vi "Sudoku Solver.vi"(10 "Board":i32[][](array[numeric])=[[0, 0, 0, 0, 0, 0, 0, 0, 0], [0, 0, 0, 0, 0, 0, 0, 0, 0], [0, 0, 0, 0, 0, 0, 0, 0, 0], [0, 0, 0, 0, 0, 0, 0, 0, 0], [0, 0, 0, 0, 0, 0, 0, 0, 0], [0, 0, 0, 0, 0, 0, 0, 0, 0], [0, 0, 0, 0, 0, 0, 0, 0, 0], [0, 0, 0, 0, 0, 0, 0, 0, 0], [0, 0, 0, 0, 0, 0, 0, 0, 0]]) -> (1 "Solved":bool=TRUE, 3 "Sudoku Solution":i32[][](array[numeric])=[[4, 3, 5, 2, 6, 9, 7, 8, 1], [6, 8, 2, 5, 7, 1, 4, 9, 3], [1, 9, 7, 8, 3, 4, 5, 6, 2], [8, 2, 6, 1, 9, 5, 3, 4, 7], [3, 7, 4, 6, 8, 2, 9, 1, 5], [9, 5, 1, 7, 4, 3, 6, 2, 8], [5, 1, 9, 3, 2, 6, 8, 7, 4], [2, 4, 8, 9, 5, 7, 1, 3, 6], [7, 6, 3, 4, 1, 8, 2, 5, 9]])   [LabVIEW 2023]
doc: "Main VI of Sudoku Solver. \n\nInputs\n- Board: Input of Board Configuration\n- Current Cell: Row and Column of Current Cell\n\nOutputs\n- Sudoku Solution: Current Board Configuration\n- Solved: TRUE if Sudoku is solved"
panel:
  # "Instructions:\n1. Input your Sudoku in \"Board\". \"0\" represents empty cells.\n2. Run VI to solve the Sudoku"
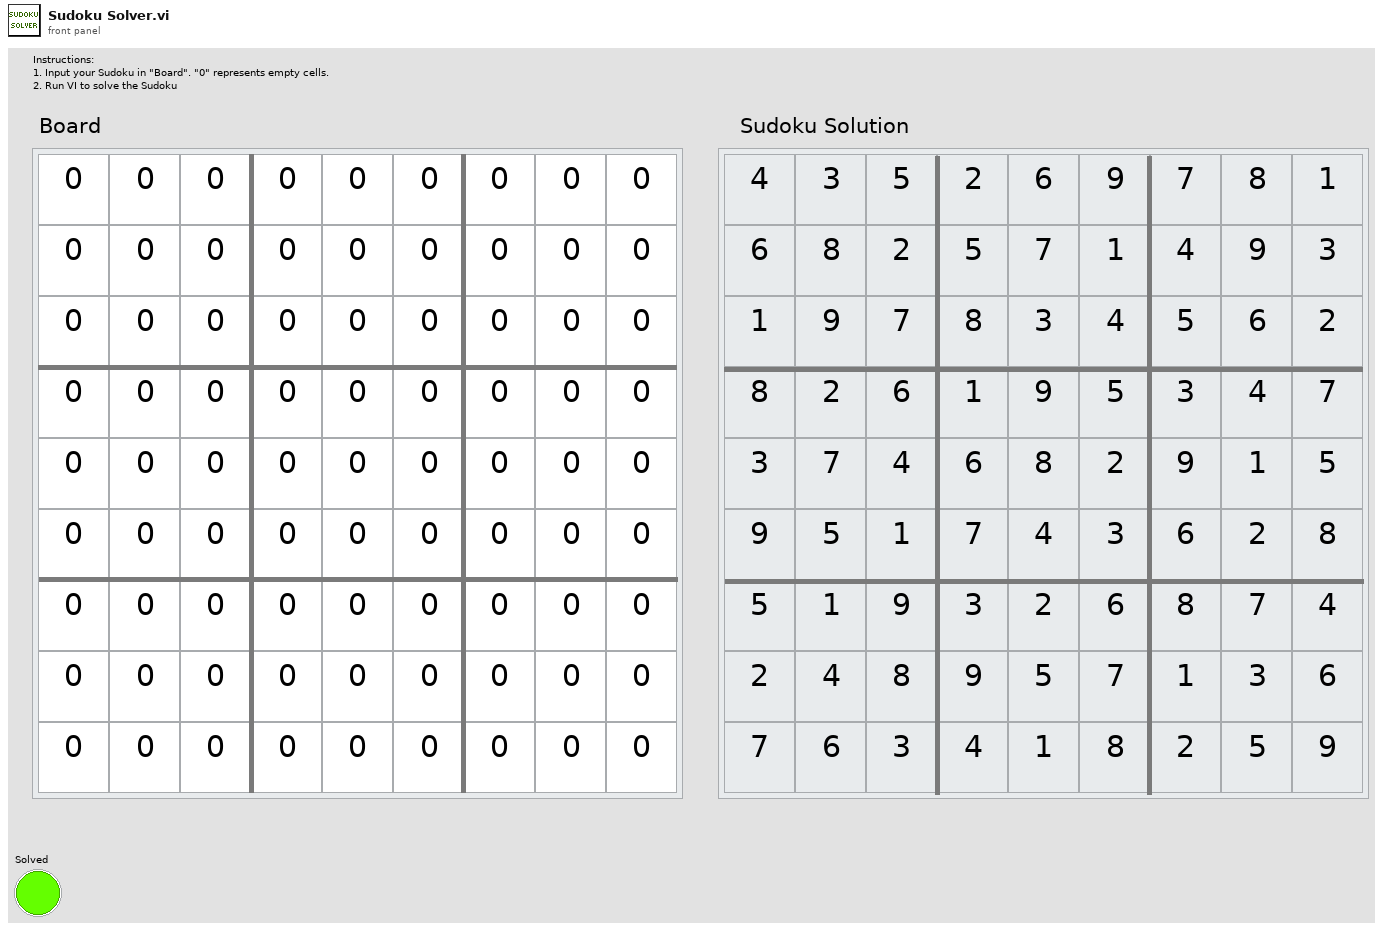
[diagram p1: front panel]
types:
  T1 = typedef "CurrentCell.ctl" = cluster{"Row":i32, "Column":i32}
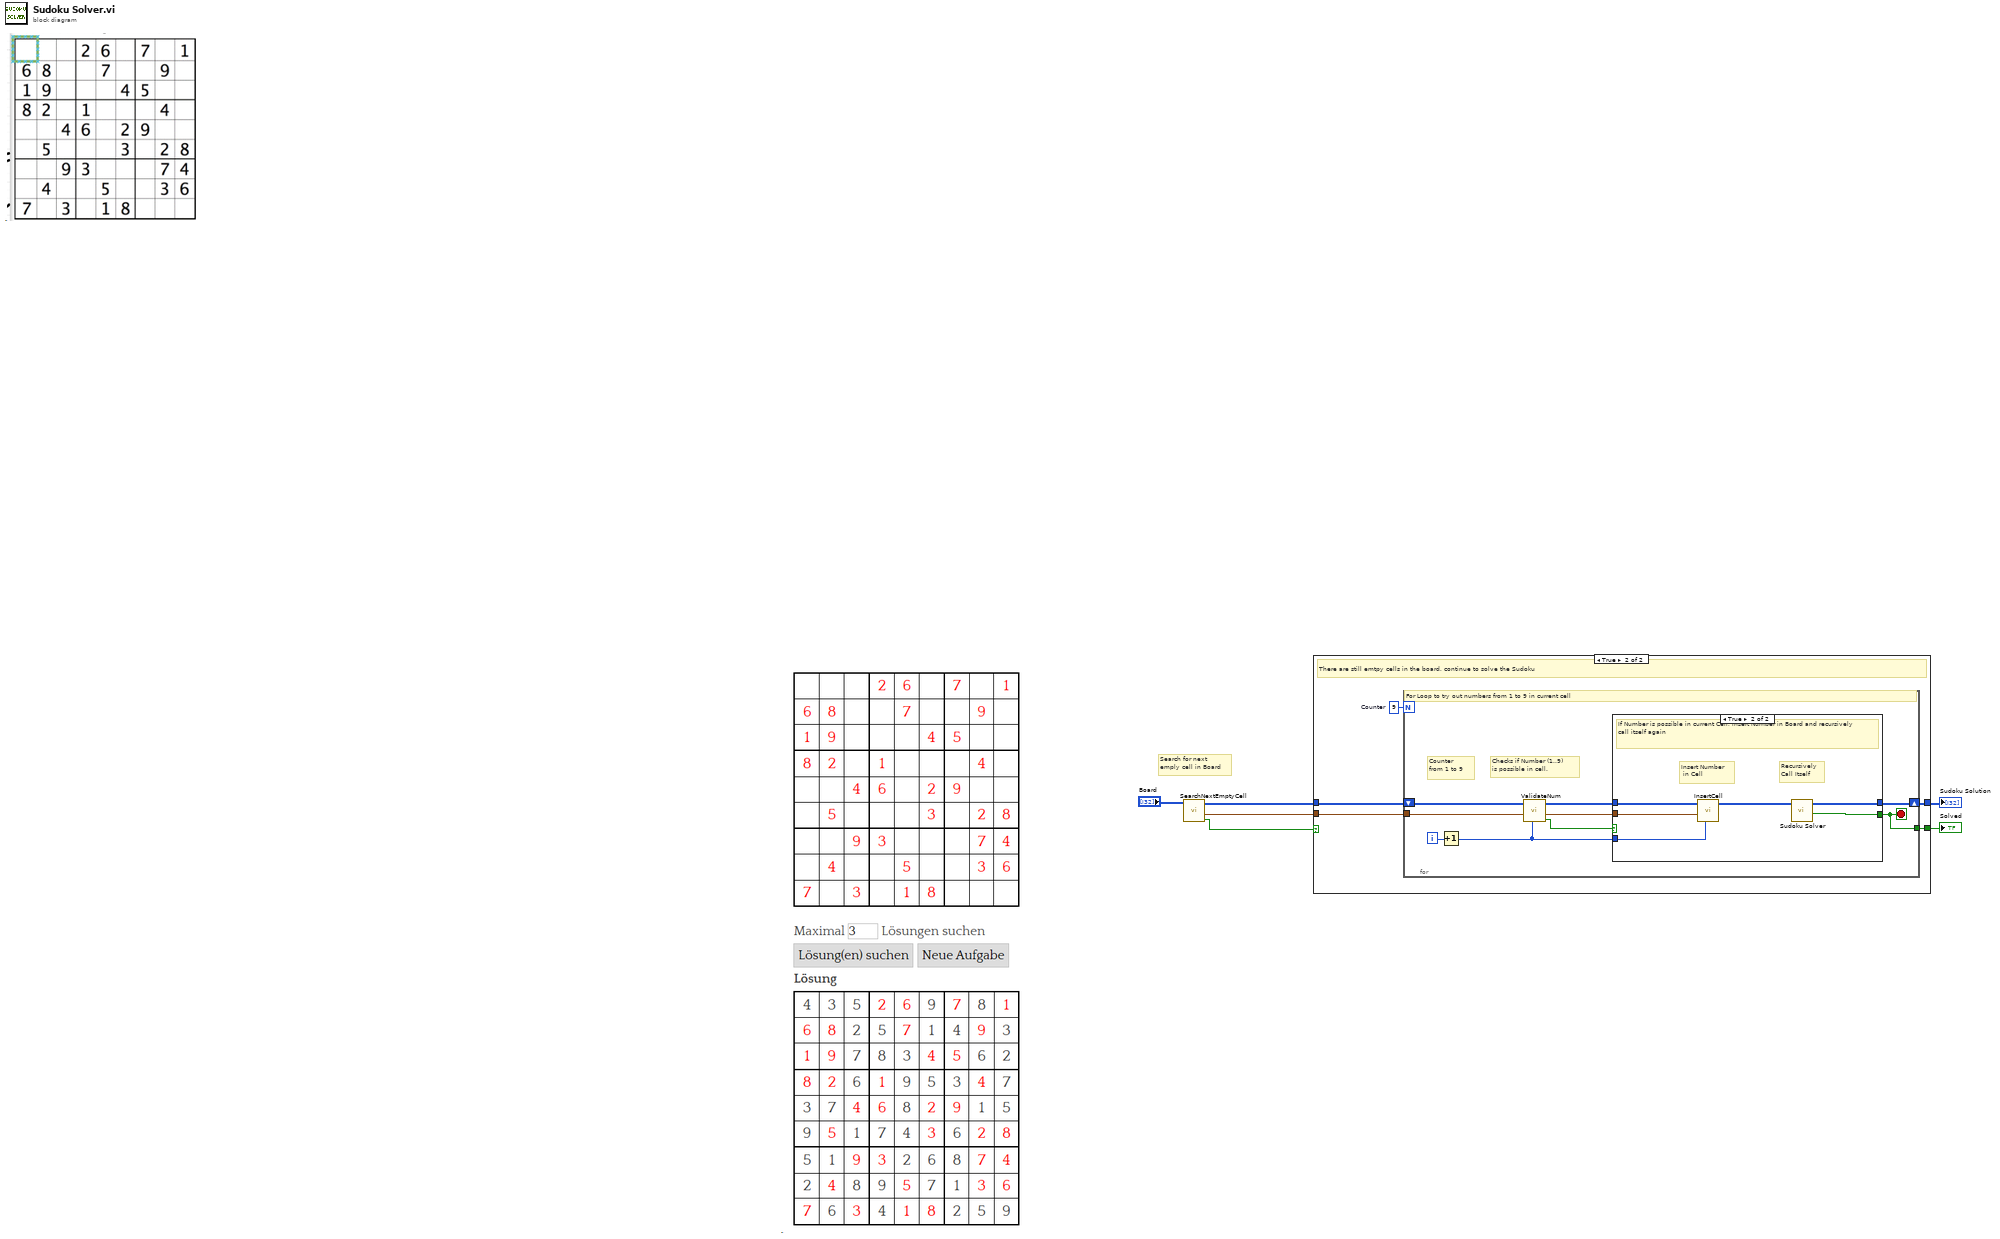
[diagram p0: block diagram]
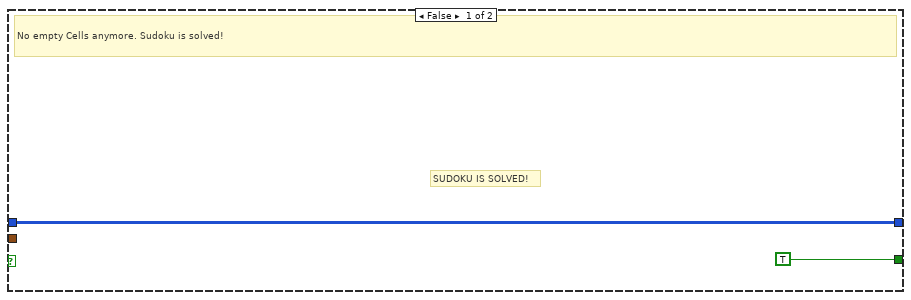
[diagram p2: hidden frame]
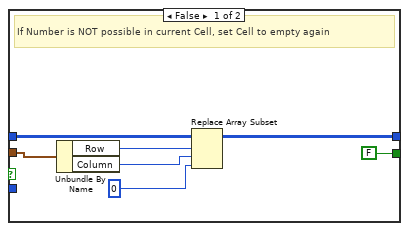
[diagram p3: hidden frame]
diagram:
  # "Search for next \nemply cell in Board"
  n1 = call "SearchNextEmptyCell.vi"("Board"="Board") -> ("empty Cell found?"=w3:bool, "Cell"=w1:T1, "Board"=w2:i32[][])  [unwired: 8 in]
  n2 = case shown="True" w3 {
    tunnel: [w7 w12] -> w4
    tunnel: [TRUE w11] -> w5
    tunnel: w2 -> [w7 w10]
    tunnel: w1 -> [_ w9]
    frame False {
      # "SUDOKU IS SOLVED!"
      # "No empty Cells anymore. Sudoku is solved!"
    }
    frame True {
      w13 = 9  # Counter
      # "There are still emtpy cells in the board, continue to solve the Sudoku"
      n3 = for {
        N: w13 -> [_]
        tunnel: [w20] -> w11
        shift-right: [w21] -> w12
        shift-left: w10 -> [w19]
        tunnel: w9 -> [w16]
        i -> [w22]
        stop <- w20 stop-if-true
        # "Checks if Number (1..9)\nis possible in cell."
        # "Counter \nfrom 1 to 9"
        # "For Loop to try out numbers from 1 to 9 in current cell"
        n4 = Increment(x=w22) -> (x+1=w14:i32)
        n5 = call "ValidateNum.vi"("Number"=w14, "Current Cell"=w16, "Board"=w19) -> ("Valid?"=w15:bool, "Current Cell"=w17:T1, "Board"=w18:i32[][])  [unwired: 6 in]
        n6 = case shown="True" w15 {
          tunnel: w18 -> [w28 w35]
          tunnel: w17 -> [w25 w34]
          tunnel: [w27 w33] -> w21
          tunnel: [FALSE ("Solved?") w31] -> w20
          tunnel: w14 -> [_ w30]
          frame False {
            # "If Number is NOT possible in current Cell, set Cell to empty again"
            n7 = Unbundle By Name(w25) -> ("Row"=w24:i32, "Column"=w23:i32)
            n8 = Replace Array Subset(array=w28, new element=0 ("new element/subarray"), index (row)=w24, index (col)=w23) -> (w27:i32[][])
          }
          frame True {
            # "Recursively \nCall Itself"
            # "Insert Number\n in Cell"
            # "If Number is possible in current Cell, insert Number in Board and recursively call itself again"
            n9 = call "InsertCell.vi"("Number"=w30, "Current Cell"=w34, "Board"=w35) -> ("Board"=w32:i32[][])  [unwired: 8 in]
            n10 = call "Sudoku Solver.vi"("Board"=w32) -> ("Solved"=w31:bool, "Sudoku Solution"=w33:i32[][])  [unwired: 8 in]
          }
        }
      }
    }
  }
  "Solved" <- w5
  "Sudoku Solution" <- w4
